vi "Initialise.vi"(11 "Size":u16 format="%04x") -> (3 "Memory out":refnum<class "Memory.lvclass">)   [LabVIEW 2021, in "Memory.lvclass"]
uses:
  Memory.lvclass
  Memory.lvclass/Memory.ctl
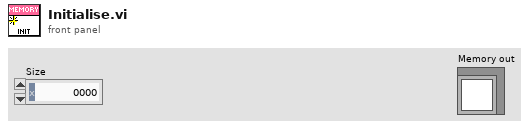
[diagram p1: front panel]
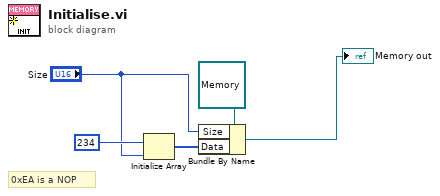
[diagram p0: block diagram]
diagram:
  # "0xEA is a NOP"
  n1 = Initialize Array(u8 234 ("element"), "Size") -> (w3:u8[])
  n2 = Bundle By Name(cluster=refnum<class "Memory.lvclass"> refnum ("EEPROM in"), "Size"="Size", "Data"=w3) -> (→"Memory out":refnum<class "Memory.lvclass">)
